vi "Open_Fast_Manual.vi"(4 "Error IN Toolkit":i32, 5 "Error IN LabVIEW":errorcluster, 6 "Radio":i32, 8 "blocks":i32, 10 "threads":i32) -> (18 "Error OUT Toolkit":i32, 19 "Error OUT LabVIEW":errorcluster)   [LabVIEW 2018]
doc: "Algorithm used to eliminate small holes within white regions (zones with 1). Applies to a \"Dilate\" algorithm and later to \"Erode\". It receives the number of threads and blocks for the GPU and the radio for the size of the kernel that is applied to the process.\n\nFor correct operation it should receives an error that comes from a VI of some processing algorithm or that contains a copy data of CPU-GPU."
uses:
  dll/LibreriaAutis_3.dll
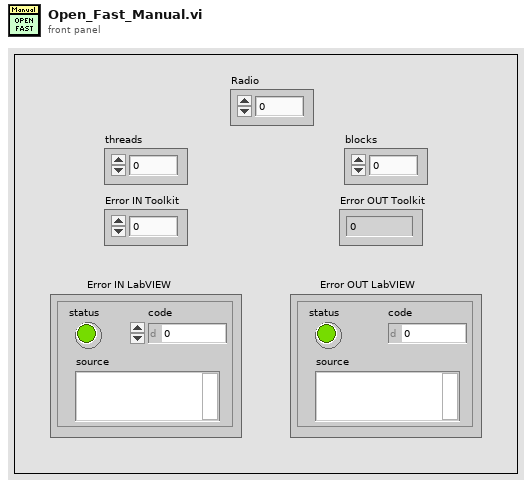
[diagram p1: front panel]
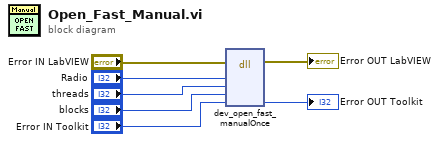
[diagram p0: block diagram]
diagram:
  n1 = dll-call lib="C:/Users/AUTIS/Desktop/LibreriaAUTIS/LabVIEW/dll/LibreriaAutis_3.dll" fn="dev_open_fast_manualOnce"(error in="Error IN LabVIEW", "radio"="Radio", "threads"="threads", "blocks"="blocks", "error"="Error IN Toolkit") -> (error out=→"Error OUT LabVIEW":errorcluster, "error"=→"Error OUT Toolkit":i32)  [unwired: 6 in, 1 out]
